vi "Write (Value).vi"(8 "error in (no error)":errorcluster, 10 "Value":variant, 11 "State in":refnum<class "State.lvclass">) -> (0 "error out":errorcluster, 3 "State out":refnum<class "State.lvclass">)   [LabVIEW 2017, in "Promise Future.lvlib" / "State.lvclass"]
uses:
  State.lvclass
  State.lvclass/State.ctl
  <vilib>/Utility/error.llb/Error Cluster From Error Code.vi
  <vilib>/ErrorRing/Error Ring.xnode
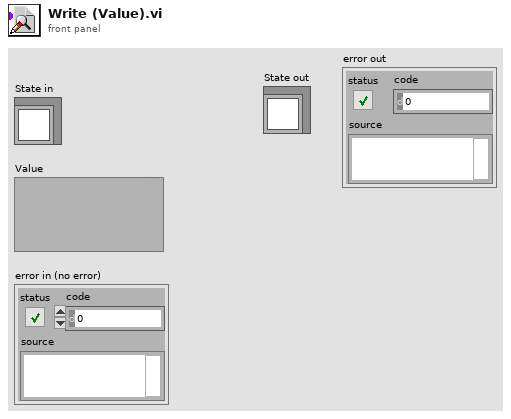
[diagram p1: front panel]
types:
  T1 = typedef "Promise.lvlib/State.lvclass/State Core.ctl" = cluster{"Value":refnum<queue>, "Callbacks":refnum<queue>, "Semaphore":T2}
  T2 = typedef "Semaphore RefNum" = refnum<k1>
  T3 = cluster{"Value":variant, "error in (no error)":errorcluster}
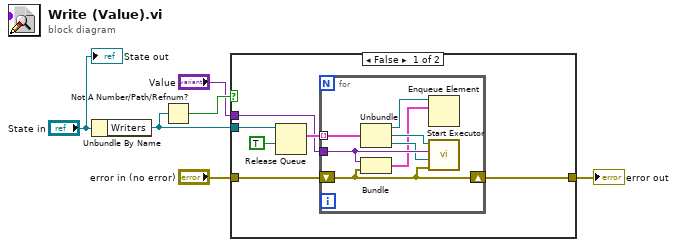
[diagram p0: block diagram]
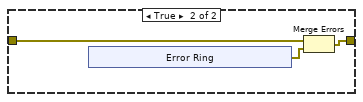
[diagram p2: hidden frame]
diagram:
  n1 = Unbundle By Name("State in") -> ("Writers"=w2:refnum<queue>)
  n2 = Not A Number/Path/Refnum?(number/path/refnum=w2) -> (NaN/Path/Refnum?=w5:bool)
  n3 = case shown="False" w5 {
    tunnel: "error in (no error)" -> [w9 w22]
    tunnel: [w8 w21] -> w6
    tunnel: "Value" -> [w10 _]
    tunnel: w2 -> [w7 _]
    frame False {
      n4 = Release Queue(queue=w7, force destroy? (F)=TRUE) -> (remaining elements=w12:T1[])  [unwired: 1 in, 2 out]
      n5 = for {
        tunnel: w12 -> [w19] mode=indexing
        tunnel: w10 -> [w17]
        shift-right: [w15] -> w8
        shift-left: w9 -> [w15]
        n6 = Unbundle(w19) -> ("Value"=w16:refnum<queue>, "Callbacks"=w18:refnum<queue>, "Semaphore"=w14:T2)
        n7 = Bundle("Value"=w17, "error in (no error)"=w15) -> (w13:T3)  [unwired: 1 in]
        n8 = Enqueue Element(queue=w16, element=w13) -> ()  [unwired: 2 in, 3 out]
        n9 = call "Start Executor.vi"("error in (no error)"=w15, "semaphore"=w14, "Value"=w17, "Callbacks"=w18) -> ()  [unwired: 8 in]
      }
    }
    frame True {
      n10 = xnode "Error Ring"() -> ("error out"=w20:errorcluster)
      n11 = Merge Errors(w22, w20) -> (w21:errorcluster)
    }
  }
  "error out" <- w6
  "State out" <- "State in"
